vi "select popup.vi"(10 "Column":i32, 11 "Popups":cluster{"Referens":refnum<vi>, "Column":i32}[](array[cluster])) -> (3 "Ring输出":refnum<vi>)   [LabVIEW 2017, in "Popup.lvclass"]
uses:
  Popup.lvclass
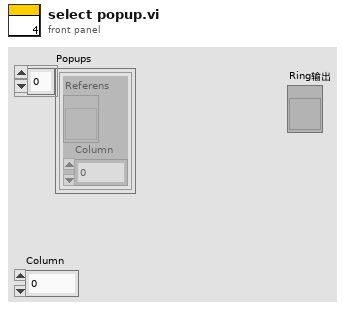
[diagram p1: front panel]
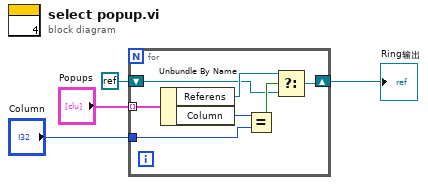
[diagram p0: block diagram]
diagram:
  n1 = for {
    tunnel: "Popups" -> [w11] mode=indexing
    tunnel: "Column" -> [w9]
    shift-right: [w5] -> w1
    shift-left: refnum<k0> refnum -> [w6]
    n2 = Unbundle By Name(w11) -> ("Referens"=w8:refnum<vi>, "Column"=w10:i32)
    n3 = Equal?(x=w10, y=w9) -> (x = y?=w7:bool)
    n4 = Select(t=w8, s=w7, f=w6) -> (s? t:f=w5:refnum<vi>)
  }
  "Ring输出" <- w1
